vi "TPNT_SendMail.vi"(4 "labmail":bool, 5 "mailserver":string="localhost", 6 "alarm message":string, 7 "application name":string, 8 "arguments":string, 9 "device":string, 10 "next alarm (msec)":i32) -> ()   [LabVIEW 2016]
uses:
  <vilib>/Utility/SMTP/NI_SMTPEmail.lvlib
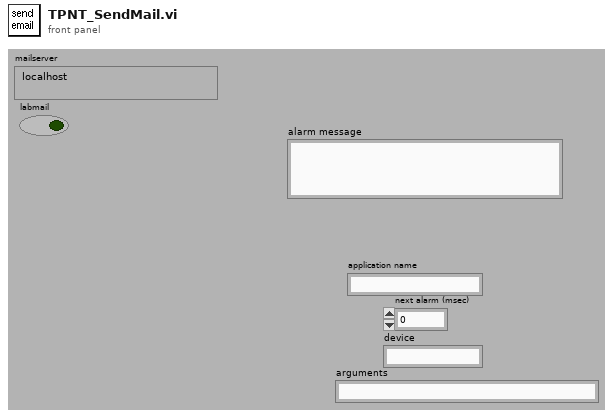
[diagram p1: front panel]
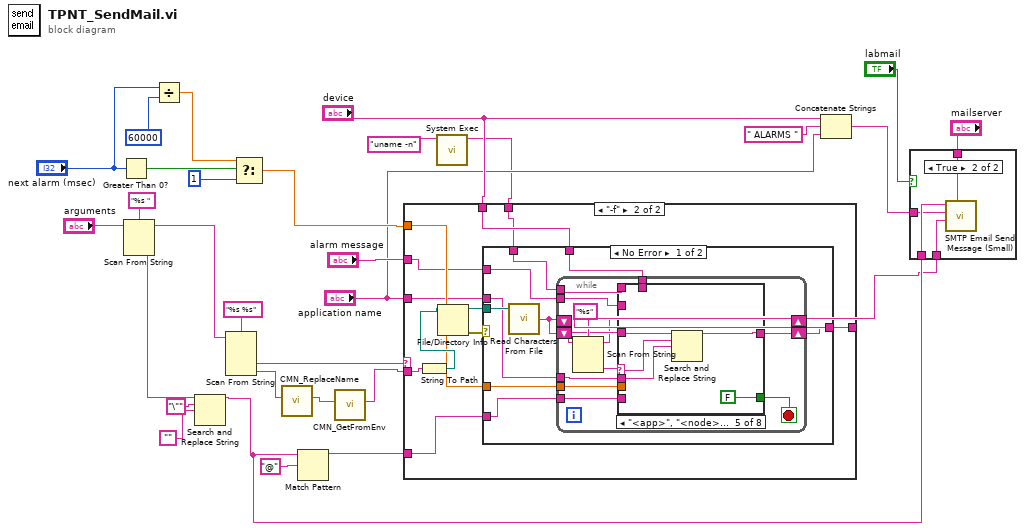
[diagram p0: block diagram]
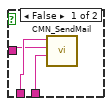
[diagram p2: hidden frame]
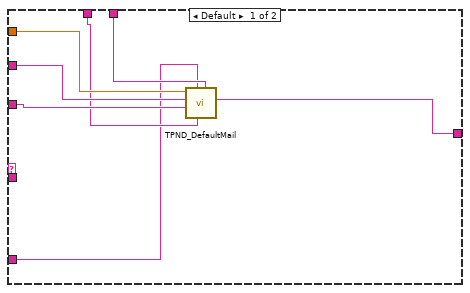
[diagram p3: hidden frame]
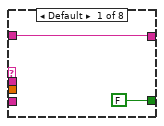
[diagram p4: hidden frame]
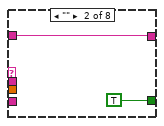
[diagram p5: hidden frame]
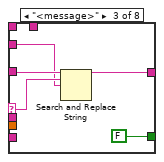
[diagram p6: hidden frame]
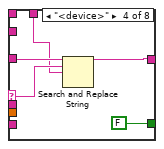
[diagram p7: hidden frame]
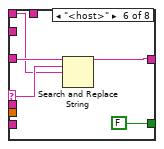
[diagram p8: hidden frame]
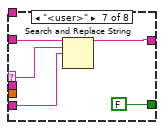
[diagram p9: hidden frame]
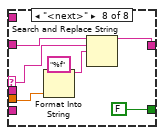
[diagram p10: hidden frame]
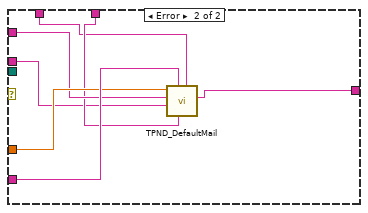
[diagram p11: hidden frame]
diagram:
  n1 = Greater Than 0?(x="next alarm (msec)") -> (x > 0?=w17:bool)
  n2 = Scan From String(format string="%s ", input string="arguments") -> (remaining string=w24:string, output 1=w19:string)  [unwired: 2 in, 3 out]
  n3 = Divide(x="next alarm (msec)", y=60000) -> (x/y=w26:dbl)
  n4 = Search and Replace String(input string=w19, search string="\"", replace string="") -> (result string=w15:string)  [unwired: 1 in, 7 out]
  n5 = Scan From String(format string="%s %s", input string=w24) -> (output 1=w22:string, output 2=w2:string)  [unwired: 2 in, 5 out]
  n6 = Select(t=w26, s=w17, f=1) -> (s? t:f=w21:dbl)
  n7 = call "CMN_ReplaceName.vi"("name in"=w2) -> ("name out"=w1:string)  [unwired: 1 in, 9 out]
  n8 = Match Pattern(string=w15, regular expression="@") -> (before substring=w6:string)  [unwired: 4 out]
  n9 = call "CMN_GetFromEnv.vi"("str in"=w1) -> ("str out"=w12:string)  [unwired: 10 out]
  n10 = call <vilib>:"System Exec.vi"("command line"="uname -n") -> ("standard output"=w3:string)  [unwired: 5 in, 5 out]
  n11 = case shown="\"-f\"" w22 {
    tunnel: w12 -> [_ w48]
    tunnel: [w37 w43] -> w13
    tunnel: w21 -> [w35 w44]
    tunnel: w3 -> [w36 w38]
    tunnel: "alarm message" -> [w34 w42]
    tunnel: "device" -> [w32 w41]
    tunnel: "application name" -> [w33 w39]
    tunnel: w6 -> [w31 w40]
    frame Default {
      n12 = call "TPND_DefaultMail.vi"("host name"=w36, "device"=w32, "user"=w31, "application name"=w33, "alarm message"=w34, "next alarm"=w35) -> ("mail out"=w37:string)  [unwired: 5 out]
    }
    frame "-f" {
      n13 = String To Path(string=w48) -> (path=w47:path)
      n14 = File/Directory Info(path=w47) -> (path out=w45:path, error out=w46:errorcluster)  [unwired: 1 in, 5 out]
      n15 = case shown="No Error" w46 {
        tunnel: w45 -> [w57 _]
        tunnel: [w54 w107] -> w43
        tunnel: w44 -> [w55 w112]
        tunnel: w42 -> [w52 w111]
        tunnel: w41 -> [w53 w110]
        tunnel: w40 -> [w50 w113]
        tunnel: w39 -> [w49 w109]
        tunnel: w38 -> [w51 w108]
        frame No Error {
          n16 = call <vilib>:"Read Characters From File.vi"("file path (dialog if empty)"=w57) -> ("character string"=w56:string)  [unwired: 1 in, 7 out]
          n17 = while {
            shift-right: [w65] -> _
            shift-left: w56 -> [w70]
            shift-right: [w66] -> w54
            shift-left: w56 -> [w67]
            tunnel: w55 -> [w64]
            tunnel: w53 -> [w63]
            tunnel: w52 -> [w61]
            tunnel: w51 -> [w60]
            tunnel: w50 -> [w59]
            tunnel: w49 -> [w58]
            stop <- w62 stop-if-true
            n18 = Scan From String(format string="%s", input string=w70) -> (remaining string=w65:string, output 1=w68:string)  [unwired: 2 in, 3 out]
            n19 = case shown="\"<app>\", \"<node>\"" w68 {
              selector: w68 -> [_ _ w77 w82 w87 w92 w97 w102]
              tunnel: w67 -> [w72 w74 w78 w83 w88 w93 w98 w103]
              tunnel: [w72 w74 w76 w80 w86 w91 w96 w100] -> w66
              tunnel: w64 -> [_ _ _ _ _ _ _ w105]
              tunnel: w63 -> [_ _ _ w81 _ _ _ _]
              tunnel: [FALSE TRUE FALSE FALSE FALSE FALSE FALSE FALSE] -> w62
              tunnel: w61 -> [_ _ w75 _ _ _ _ _]
              tunnel: w60 -> [_ _ _ _ _ w90 _ _]
              tunnel: w59 -> [_ _ _ _ _ _ w95 _]
              tunnel: w58 -> [_ _ _ _ w85 _ _ _]
              frame Default {
              }
              frame "" {
              }
              frame "<message>" {
                n20 = Search and Replace String(input string=w78, search string=w77, replace string=w75) -> (result string=w76:string)  [unwired: 1 in, 7 out]
              }
              frame "<device>" {
                n21 = Search and Replace String(input string=w83, search string=w82, replace string=w81) -> (result string=w80:string)  [unwired: 1 in, 7 out]
              }
              frame "<app>", "<node>" {
                n22 = Search and Replace String(input string=w88, search string=w87, replace string=w85) -> (result string=w86:string)  [unwired: 1 in, 7 out]
              }
              frame "<host>" {
                n23 = Search and Replace String(input string=w93, search string=w92, replace string=w90) -> (result string=w91:string)  [unwired: 1 in, 7 out]
              }
              frame "<user>" {
                n24 = Search and Replace String(input string=w98, search string=w97, replace string=w95) -> (result string=w96:string)  [unwired: 1 in, 7 out]
              }
              frame "<next>" {
                n25 = Format Into String(format string="%f", w105) -> (resulting string=w101:string)  [unwired: 2 in, 1 out]
                n26 = Search and Replace String(input string=w103, search string=w102, replace string=w101) -> (result string=w100:string)  [unwired: 1 in, 7 out]
              }
            }
          }
        }
        frame Error {
          n27 = call "TPND_DefaultMail.vi"("host name"=w108, "device"=w110, "user"=w113, "application name"=w109, "alarm message"=w111, "next alarm"=w112) -> ("mail out"=w107:string)  [unwired: 5 out]
        }
      }
    }
  }
  n28 = Concatenate Strings("device", " ALARMS " ("string"), "application name") -> (w14:string)
  n29 = case shown="True" "labmail" {
    tunnel: w15 -> [w116 w120]
    tunnel: w14 -> [w115 w119]
    tunnel: w13 -> [w114 w118]
    tunnel: "mailserver" -> [_ w117]
    frame False {
      n30 = call "CMN_SendMail.vi"("body"=w114, "subject"=w115, "address"=w116) -> ()  [unwired: 2 in, 7 out]
    }
    frame True {
      n31 = call <vilib>:"SMTP Email Send Message (Small).vi"("mail server"=w117, "message"=w118, "subject ([No Subject])"=w119, "recipient"=w120) -> ()  [unwired: 2 in, 6 out]
    }
  }
